vi "Host_8840_1.vi"() -> ()   [LabVIEW 2019]
panel:
  out "FH:DriveFa":bool
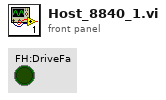
[diagram p1: front panel]
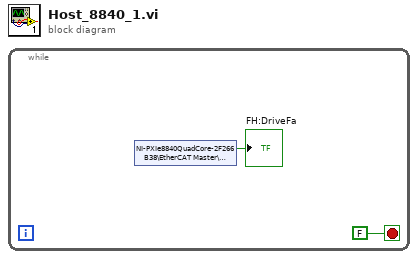
[diagram p0: block diagram]
diagram:
  n1 = while {
    stop <- FALSE stop-if-true
    n2 = shared-variable "NI-PXIe8840QuadCore-2F266B38\\EtherCAT Master\\Device\\User-Defined Variables\\FH:DriveFa"() -> (→"FH:DriveFa":bool)  [unwired: 1 in, 1 out]
  }
